vi "Open Legacy TDMS Files.vi"(0 "serial input channel":string, 5 "base tdms file path":path, 7 "file operation type":T1(ring)=enum."open (read-only)", 11 "error in (no error)":errorcluster) -> (4 "data file ref":refnum<k34>, 6 "sizes file ref":refnum<k34>, 8 "timestamp file ref":refnum<k34>, 15 "error out":errorcluster)   [LabVIEW 2023, in "GettingStarted_Common_148X_Host.lvlib"]
uses:
  GettingStarted_Common_148X_Host.lvlib
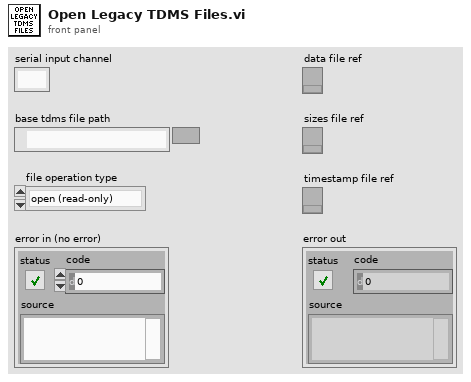
[diagram p1: front panel]
types:
  T1 = enum16{"open", "open or create", "create or replace", "create", "open (read-only)"}
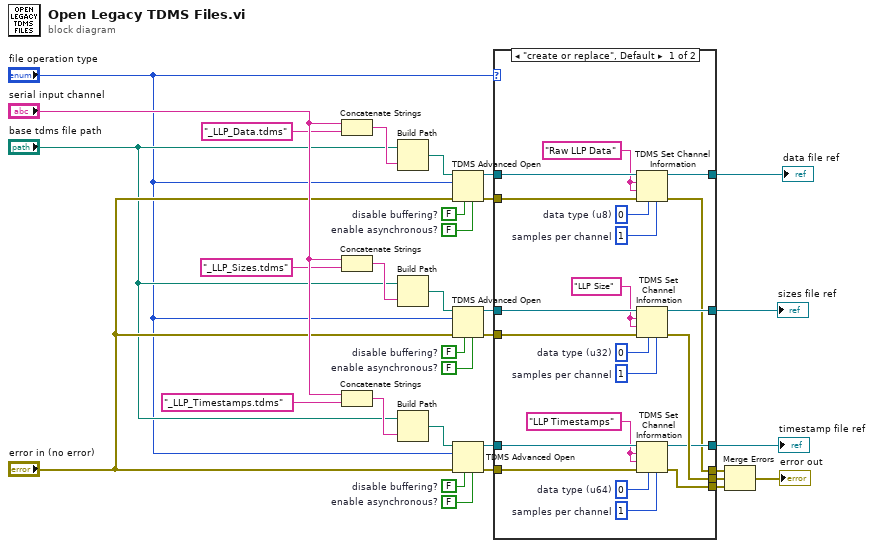
[diagram p0: block diagram]
diagram:
  w2 = FALSE  # enable asynchronous?
  w3 = FALSE  # disable buffering?
  w4 = FALSE  # enable asynchronous?
  w5 = FALSE  # disable buffering?
  w6 = FALSE  # enable asynchronous?
  w7 = FALSE  # disable buffering?
  n1 = Concatenate Strings("serial input channel", "_LLP_Data.tdms") -> (w30:string)
  n2 = Concatenate Strings("serial input channel", "_LLP_Sizes.tdms") -> (w25:string)
  n3 = Concatenate Strings("serial input channel", "_LLP_Timestamps.tdms") -> (w24:string)
  n4 = Build Path(base path="base tdms file path", name or relative path=w30) -> (appended path=w29:path)
  n5 = Build Path(base path="base tdms file path", name or relative path=w25) -> (appended path=w26:path)
  n6 = Build Path(base path="base tdms file path", name or relative path=w24) -> (appended path=w23:path)
  n7 = TDMS Advanced Open(4:w6, 6:w7, 8:"error in (no error)", 10:"file operation type", 11:w29) -> (0:w11:errorcluster, 3:w9:refnum<k34>)  [unwired: 1 out]
  n8 = TDMS Advanced Open(4:w4, 6:w5, 8:"error in (no error)", 10:"file operation type", 11:w26) -> (0:w18:errorcluster, 3:w19:refnum<k34>)  [unwired: 1 out]
  n9 = TDMS Advanced Open(4:w2, 6:w3, 8:"error in (no error)", 10:"file operation type", 11:w23) -> (0:w14:errorcluster, 3:w15:refnum<k34>)  [unwired: 1 out]
  n10 = case shown="\"create or replace\", Default" "file operation type" {
    tunnel: w19 -> [w53 w58]
    tunnel: w18 -> [w52 w55]
    tunnel: [w51 w55] -> w17
    tunnel: [w50 w58] -> w16
    tunnel: w15 -> [w48 w57]
    tunnel: w14 -> [w47 w56]
    tunnel: [w46 w56] -> w13
    tunnel: [w45 w57] -> w12
    tunnel: w11 -> [w43 w54]
    tunnel: [w42 w54] -> w10
    tunnel: w9 -> [w41 w59]
    tunnel: [w40 w59] -> w8
    frame "create or replace", Default {
      w33 = u32 1  # samples per channel
      w34 = u64 0  # data type (u64)
      w36 = u32 1  # samples per channel
      w35 = u32 0  # data type (u32)
      w37 = u32 1  # samples per channel
      w38 = u8 0  # data type (u8)
      w39 = "Raw LLP Data" ("channel and group name")
      w49 = "LLP Size" ("channel and group name")
      w44 = "LLP Timestamps" ("channel and group name")
      n11 = TDMS Set Channel Information(4:w37, 6:w38, 8:w43, 9:w39, 10:w39, 11:w41) -> (0:w42:errorcluster, 3:w40:refnum<k34>)  [unwired: 1 in]
      n12 = TDMS Set Channel Information(4:w36, 6:w35, 8:w52, 9:w49, 10:w49, 11:w53) -> (0:w51:errorcluster, 3:w50:refnum<k34>)  [unwired: 1 in]
      n13 = TDMS Set Channel Information(4:w33, 6:w34, 8:w47, 9:w44, 10:w44, 11:w48) -> (0:w46:errorcluster, 3:w45:refnum<k34>)  [unwired: 1 in]
    }
    frame "open (read-only)" {
    }
  }
  "data file ref" <- w8
  "sizes file ref" <- w16
  "timestamp file ref" <- w12
  n14 = Merge Errors(w10, w17, w13) -> (→"error out":errorcluster)
